vi "MT Modulate - Data Bit Extraction.vi"(2 "QAM Complexity":T1(ring), 3 "BitStream In":i32[](array[numeric])) -> (0 "Pilot BitStream":i32[](array[numeric]), 1 "Data BitStream":i32[](array[numeric]))   [LabVIEW 2018]
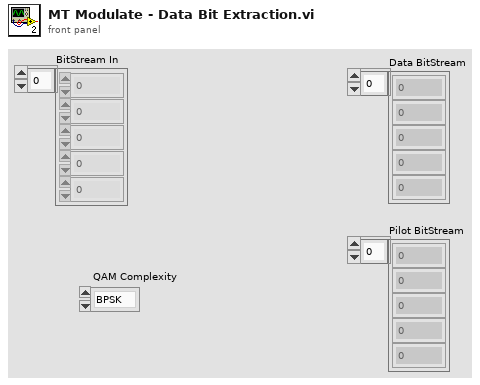
[diagram p1: front panel]
types:
  T1 = enum16{"BPSK", "QPSK", "16-QAM", "64-QAM", "256-QAM"}
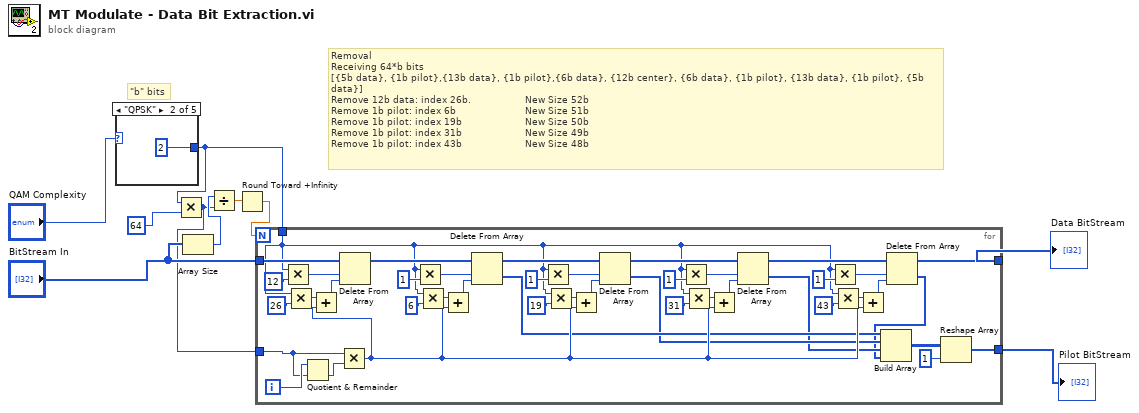
[diagram p0: block diagram]
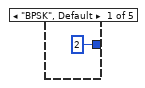
[diagram p2: hidden frame]
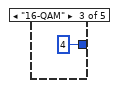
[diagram p3: hidden frame]
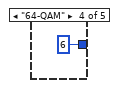
[diagram p4: hidden frame]
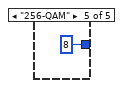
[diagram p5: hidden frame]
diagram:
  # "\"b\" bits"
  # "Removal\nReceiving 64*b bits\n[{5b data}, {1b pilot},{13b data}, {1b pilot},{6b data}, {12b center}, {6b data}, {1b pilot}, {13b data}, {1b pilot}, {5b data}]\nRemove 12b data: index 26b.                  New Size 52b\nRemove 1b pilot: index 6b                       New Size 51b  \nRemove 1b pilot: index 19b                     New Size 50b\nRemove 1b pilot: index 31b                     New Size 49b\nRemove 1b pilot: index 43b                     New Size 48b"
  n1 = case shown="\"QPSK\"" "QAM Complexity" {
    tunnel: [2 2 4 6 8] -> w8
    frame "BPSK", Default {
    }
    frame "QPSK" {
    }
    frame "16-QAM" {
    }
    frame "64-QAM" {
    }
    frame "256-QAM" {
    }
  }
  n2 = Multiply(x=w8, y=64) -> (x*y=w3:i32)
  n3 = Array Size(array="BitStream In") -> (size(s)=w7:i32)
  n4 = Divide(x=w7, y=w3) -> (x/y=w5:dbl)
  n5 = Round Toward +Infinity(x=w5) -> (ceil(x): smallest int >= x=w4:dbl)
  n6 = for {
    N: w4 -> [_]
    tunnel: "BitStream In" -> [w58]
    tunnel: w8 -> [w24]
    tunnel: w3 -> [w53]
    tunnel: [w23] -> w2
    tunnel: [w16] -> w1
    i -> [w55]
    n7 = Multiply(x=w24, y=12) -> (x*y=w57:i32)
    n8 = Multiply(x=w24, y=26) -> (x*y=w52:i32)
    n9 = Quotient & Remainder(x=w55, y=w53) -> (floor(x/y)=w54:i32)  [unwired: 1 out]
    n10 = Multiply(x=w53, y=w54) -> (x*y=w25:i32)
    n11 = Add(x=w52, y=w25) -> (x+y=w45:i32)
    n12 = Delete From Array(array=w58, length=w57, index=w45) -> (array with subset deleted=w46:i32[])  [unwired: 1 out]
    n13 = Multiply(x=w24, y=1) -> (x*y=w47:i32)
    n14 = Multiply(x=w24, y=6) -> (x*y=w49:i32)
    n15 = Add(x=w49, y=w25) -> (x+y=w44:i32)
    n16 = Delete From Array(array=w46, length=w47, index=w44) -> (deleted portion=w20:i32[], array with subset deleted=w38:i32[])
    n17 = Multiply(x=w24, y=1) -> (x*y=w42:i32)
    n18 = Multiply(x=w24, y=19) -> (x*y=w40:i32)
    n19 = Add(x=w40, y=w25) -> (x+y=w43:i32)
    n20 = Delete From Array(array=w38, length=w42, index=w43) -> (deleted portion=w19:i32[], array with subset deleted=w32:i32[])
    n21 = Multiply(x=w24, y=1) -> (x*y=w34:i32)
    n22 = Multiply(x=w24, y=31) -> (x*y=w36:i32)
    n23 = Add(x=w36, y=w25) -> (x+y=w33:i32)
    n24 = Delete From Array(array=w32, length=w34, index=w33) -> (deleted portion=w18:i32[], array with subset deleted=w26:i32[])
    n25 = Multiply(x=w24, y=1) -> (x*y=w30:i32)
    n26 = Multiply(x=w24, y=43) -> (x*y=w28:i32)
    n27 = Add(x=w28, y=w25) -> (x+y=w31:i32)
    n28 = Delete From Array(array=w26, length=w30, index=w31) -> (deleted portion=w17:i32[], array with subset deleted=w23:i32[])
    n29 = Build Array(w20, w19, w18, w17) -> (w22:i32[][])
    n30 = Reshape Array(w22, 1 ("dimension size")) -> (w16:i32[])
  }
  "Data BitStream" <- w2
  "Pilot BitStream" <- w1
